vi "VisualizeNHRDC.vi"() -> ()   [LabVIEW 2018, in "Visualization.lvlib" / "VisualizeAcPwr.lvclass"]
doc: "This VI listens for any measurement data associated with the provided PluginName and displays it to the user for analysis. The display is only suitable for data coming from the NHR Battery Simulator Plugin."
uses:
  VisualizeAcPwr.lvclass
  VisualizeBase/VisualizeBase_class/Requests/VisUserEventType.ctl
  <vilib>/event_ctls.llb/usereventprio.ctl
  AcPwr/AcPwrShared/clMeasurmentData.ctl
  <vilib>/Analysis/baseanly.llb/Mean (DBL).vi
  <extravilib>/ChannelInstances/Tag-bool/Read With Abort.vi
  <extravilib>/ChannelInstances/Tag-bool/Write With Abort.vi
  <extravilib>/ChannelInstances/Tag-bool/Instantiate.vi
  <extravilib>/ChannelInstances/Tag-bool/EndpointRead.vi
  <vilib>/Utility/error.llb/Error Cluster From Error Code.vi
  <extravilib>/ChannelInstances/Tag-bool/Endpoint.vi
  <vilib>/ErrorRing/Error Ring.xnode
  VisualizeBase/VisualizeBase_class/VisualizeBase.lvclass
  <userlib>/NIST/NISTErrorLib/NISTErrorLib.lvlib
  <vilib>/Analysis/NI_AALBase.lvlib
  AcPwr/AcPwrShared/AcPwrShared.lvlib
  <extravilib>/ChannelInstances/Tag-bool.lvlib
panel:
  in  "Tab Control":enum32{"Chart", "XY Graph"}(tab)
  out "NHRDC":waveform(dbl)[](graph)=[{"t0"=timestamp(3657200531.6397257 s since 1904-01-01), "dt"=1.0, "Y"=[46.19]}, {"t0"=timestamp(3657200531.6397257 s since 1904-01-01), "dt"=1.0, "Y"=[2.0]}, {"t0"=timestamp(3657200531.6397257 s since 1904-01-01), "dt"=1.0, "Y"=[60.0]}]
  in  "PlotYAxis":u32[](array[numeric])=[0, 1, 0] max=1
  out "Incorrect DataType?":bool
  out "Current (A)":dbl(knob) scale=0.0..15.0
  out "Voltage (V)":dbl(knob) scale=0.0..100.0
  out "XY Graph":cluster{"Current":dbl[], "Voltage":dbl[]}[](graph)
  in  "Clear Graph":bool
  in  "PluginName":string="AcPwr.NHRDC0"
  out "ErrorArray":errorcluster[](array[cluster])
  in  "btnStop":bool
  in  "btnReset":bool
  in  "btnClear":bool
  # "0=Left Axis and 1=Right Axis"
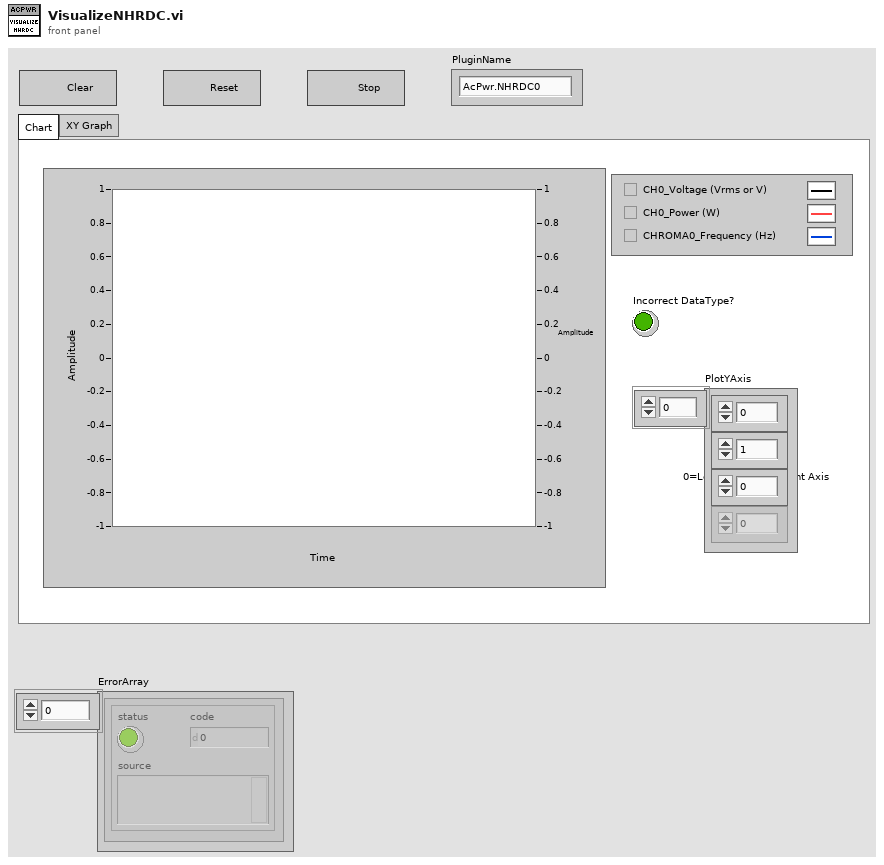
[diagram p1: front panel]
types:
  T1 = typedef "Visualization.lvlib/VisualizeBase.lvclass/VisRequestEvents.ctl" = cluster{"StopRequest":refnum<user-event>, "ResetRequest":refnum<user-event>, "FP Pop In or Out":refnum<user-event>}
  T2 = typedef "AcPwrShared.lvlib/AcPwrBroadcastEvents.ctl" = cluster{"DidInit":refnum<user-event>, "StatusUpdate":refnum<user-event>, "ErrorReport":refnum<user-event>, "DidStop":refnum<user-event>, "PathToINI":refnum<user-event>, "Measurements":refnum<user-event>, "LoadConfigFile":refnum<user-event>, "GetSettings":refnum<user-event>, "SetSettings":refnum<user-event>, "GetType&ID":refnum<user-event>, "GotSettings":refnum<user-event>}
  T3 = typedef "AcPwrShared.lvlib/clMeasurmentData.ctl" = cluster{"MeasName":string, "XML Data":string, "WaveformData":waveform(dbl)[]}
  T4 = typedef "Visualization.lvlib/VisualizeBase.lvclass/VisUserEventType.ctl" = cluster{"BusIndex":i8, "Data":variant}
  T5 = typedef "usereventprio.ctl" = enum32{"high priority", "normal priority"}
  T6 = typedef "Tag-bool.lvlib/))Channel.ctl" = refnum<queue>
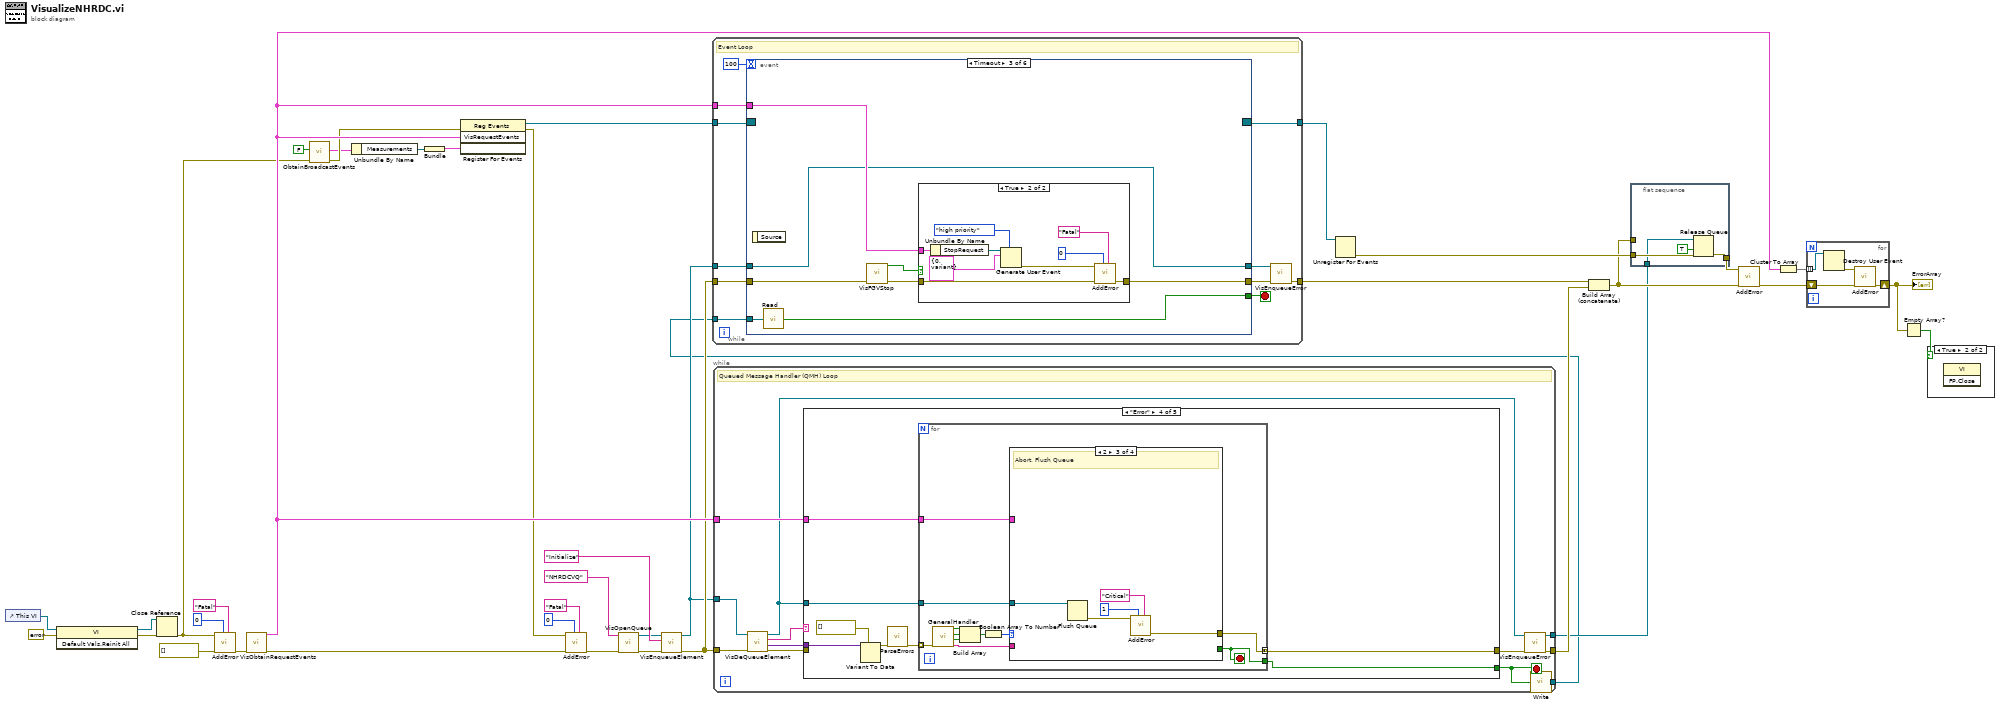
[diagram p0: block diagram]
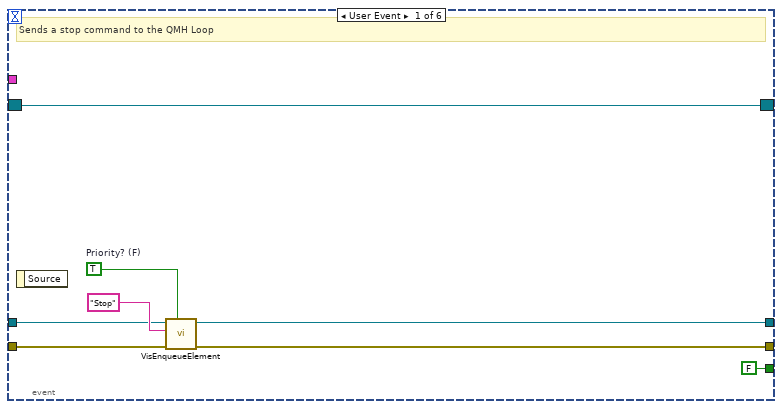
[diagram p2: hidden frame]
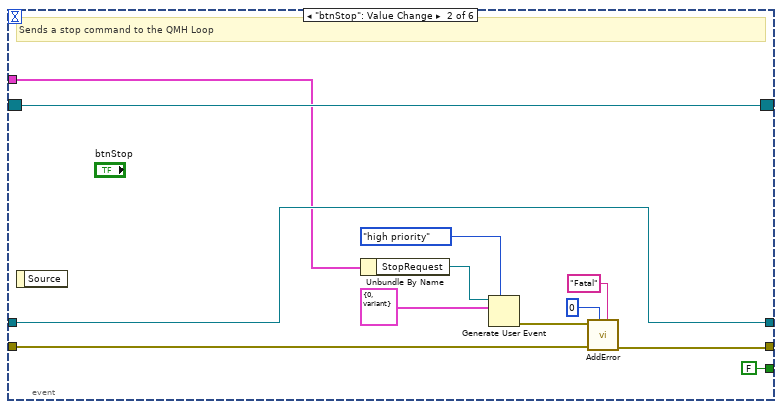
[diagram p3: hidden frame]
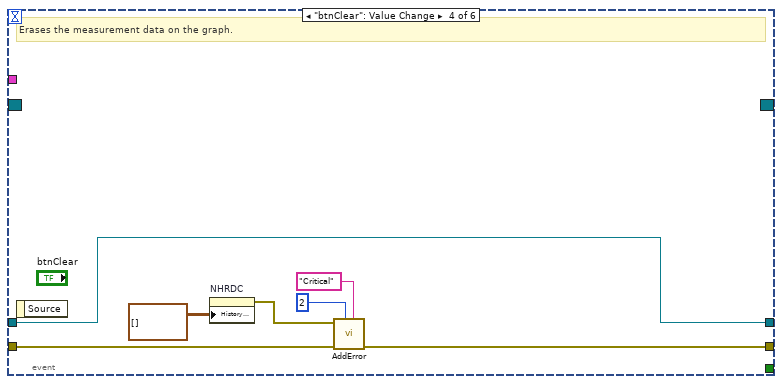
[diagram p5: hidden frame]
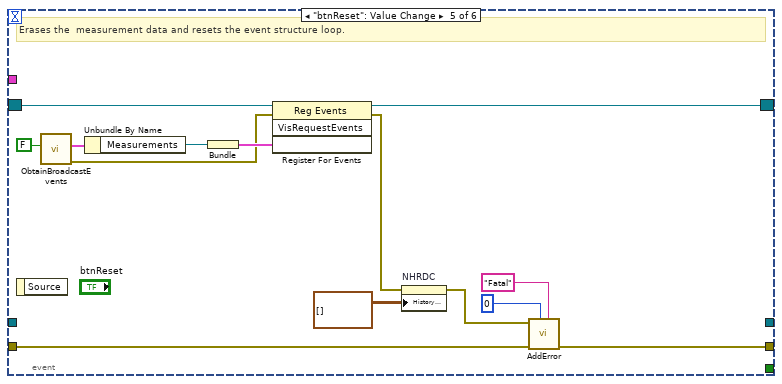
[diagram p6: hidden frame]
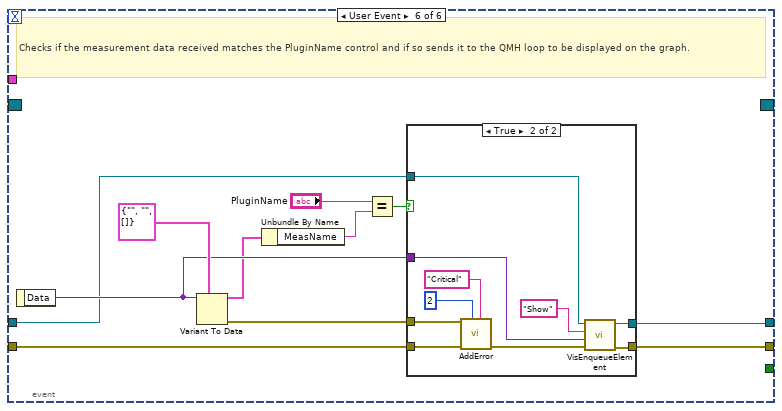
[diagram p7: hidden frame]
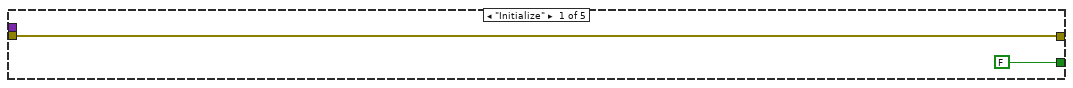
[diagram p9: hidden frame]
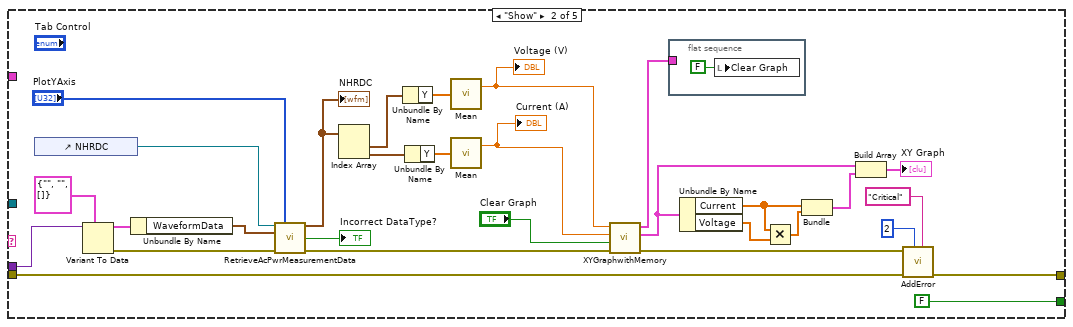
[diagram p10: hidden frame]
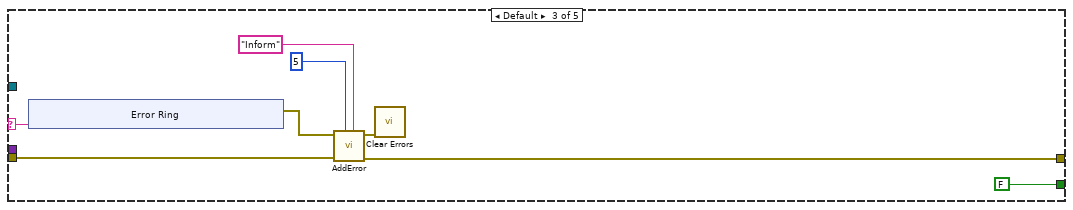
[diagram p11: hidden frame]
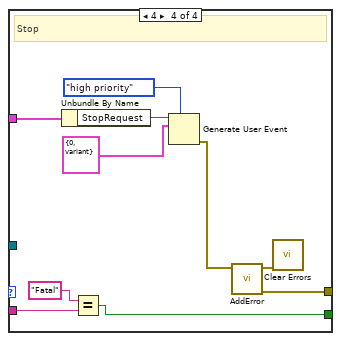
[diagram p14: hidden frame]
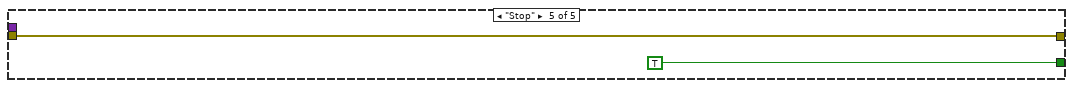
[diagram p15: hidden frame]
diagram:
  n1 = control-ref of="This VI"() -> (w26:refnum<vi>)
  n2 = invoke class="VI" method="Default Vals.Reinit All"(reference=w26, error in=errorcluster {"status"=FALSE, "code"=0, "source"=""} ("error in (no error)")) -> (reference out=w23:refnum<vi>, error out=w24:errorcluster)  [unwired: 1 in, 1 out]
  n3 = Close Reference(reference=w23, error in (no error)=w24) -> (error out=w21:errorcluster)
  n4 = call <userlib>:"AddError.vi"("Severity"="Fatal" ("String"), "Priority"=u8 0, "ErrorArray In"=errorcluster[] [] ("ErrorArray"), "error in (no error)"=w21) -> ("ErrorArray Out"=w38:errorcluster[])  [unwired: 6 in, 1 out]
  n5 = call "VisObtainRequestEvents.vi"("Error"=w38) -> ("Error"=w13:errorcluster[], "VisRequestEvents"=w30:T1)  [unwired: 9 in]
  n6 = call "ObtainBroadcastEvents.vi"("error in (no error)"=w21, "CreateNew? (F)"=FALSE) -> ("error out"=w20:errorcluster, "clAcPwrEvents"=w19:T2)  [unwired: 8 in]
  n7 = Unbundle By Name(w19) -> ("Measurements"=w28:refnum<user-event>)
  n8 = Bundle("Measurements"=w28) -> (w27:cluster{"Measurements":refnum<user-event>})  [unwired: 1 in]
  n9 = register-events(error in=w20, w30, w27) -> (reference out=w39:refnum<event-registration>, error out=w3:errorcluster)  [unwired: 1 in]
  n10 = call <userlib>:"AddError.vi"("Severity"="Fatal" ("String"), "Priority"=u8 0, "ErrorArray In"=w13, "error in (no error)"=w3) -> ("ErrorArray Out"=w10:errorcluster[])  [unwired: 6 in, 1 out]
  n11 = call "VisOpenQueue.vi"("Error Array In"=w10, "QueueName"="NHRDCVQ" ("QueuName")) -> ("Error Array Out"=w8:errorcluster[], "queue out"=w5:refnum<queue>)  [unwired: 8 in]
  n12 = call "VisEnqueueElement.vi"("Error Array In"=w8, "Message"="Initialize", "queue in"=w5) -> ("Error Array Out"=w7:errorcluster[], "queue out"=w4:refnum<queue>)  [unwired: 7 in]
  n13 = while {
    tunnel: w7 -> [w47]
    tunnel: [w49] -> w34
    tunnel: w30 -> [w48]
    tunnel: w4 -> [w46]
    tunnel: [w41] -> w2
    tunnel: [w40] -> w1
    stop <- w50 stop-if-true
    # "Queued Message Handler (QMH) Loop"
    n14 = call "VisDeQueueElement.vi"("Error Array In"=w47, "Queue In"=w46) -> ("Error Array Out"=w45:errorcluster[], "Data"=w44:variant, "Message"=w43:string, "Queue Out"=w42:refnum<queue>)  [unwired: 6 in]
    n15 = case shown="\"Error\"" w43 {
      selector: w43 -> [_ _ w92 _ _]
      tunnel: w44 -> [_ w79 _ w107 _]
      tunnel: w45 -> [w53 w80 w90 _ w134]
      tunnel: [w53 w83 w89 w103 w134] -> w51
      tunnel: [FALSE FALSE FALSE w102 TRUE] -> w50
      tunnel: w48 -> [_ _ _ w101 _]
      tunnel: w42 -> [_ _ _ w100 _]
      frame "Initialize" {
      }
      frame "Show" {
        n16 = control-ref of="NHRDC"() -> (w54:refnum<vi>)
        n17 = Variant To Data(type=T3 {"MeasName"="", "XML Data"="", "WaveformData"=[]} ("MeasurmentDataCluster"), Variant=w79) -> (data=w58:T3, error out=w61:errorcluster)  [unwired: 1 in]
        n18 = Unbundle By Name(w58) -> ("WaveformData"=w57:waveform(dbl)[])
        n19 = call "RetrieveAcPwrMeasurementData.vi"("WaveformChartReference"=w54, "PlotYScale"="PlotYAxis", "WaveformArrayIn"=w57, "error in (no error)"=w61) -> ("WaveformArrayOut"=w55:waveform(dbl)[], "Incorrect DataType?"=→"Incorrect DataType?":bool, "error out"=w60:errorcluster)  [unwired: 7 in, 2 out]
        "NHRDC" <- w55
        n20 = Index Array(array=w55) -> (element #1=w78:waveform(dbl), element #2=w77:waveform(dbl))  [unwired: 2 in]
        n21 = Unbundle By Name(w78) -> ("Y"=w75:dbl[])
        n22 = Unbundle By Name(w77) -> ("Y"=w74:dbl[])
        n23 = call-poly <vilib>:"Mean.vi"("X"=w75) -> ("mean"=w72:dbl)  [unwired: 1 out]
        "Voltage (V)" <- w72
        n24 = call-poly <vilib>:"Mean.vi"("X"=w74) -> ("mean"=w70:dbl)  [unwired: 1 out]
        "Current (A)" <- w70
        n25 = call "XYGraphwithMemory.vi"("Error In"=w60, "Clear Graph"="Clear Graph", "Current"=w70, "Voltage"=w72) -> ("Error Out"=w71:errorcluster, "output cluster"=w68:cluster{"Current":dbl[], "Voltage":dbl[]}, "Cluster"=w69:cluster{"Array":dbl[], "Array":dbl[]})  [unwired: 5 in]
        n26 = flat-sequence {
          tunnel: w69 -> [_]
          frame #0 {
            n27 = local write "Clear Graph"(FALSE ("Clear Graph")) -> ()
          }
        }
        n28 = Unbundle By Name(w68) -> ("Current"=w64:dbl[], "Voltage"=w65:dbl[])
        n29 = Multiply(x=w64, y=w65) -> (x*y=w63:dbl[])
        n30 = Bundle("Current"=w64, w63) -> (w66:cluster{"Current":dbl[], dbl[]})  [unwired: 1 in]
        n31 = Build Array(w68, w66) -> (→"XY Graph":cluster{"Current":dbl[], "Voltage":dbl[]}[])
        n32 = call <userlib>:"AddError.vi"("Severity"="Critical" ("String"), "Priority"=u8 2, "ErrorArray In"=w80, "error in (no error)"=w71) -> ("ErrorArray Out"=w83:errorcluster[])  [unwired: 6 in, 1 out]
      }
      frame Default {
        n33 = xnode "Error Ring"("parameter 0"=w92) -> ("error out"=w91:errorcluster)
        n34 = call <userlib>:"AddError.vi"("Severity"="Inform" ("String"), "Priority"=u8 5, "ErrorArray In"=w90, "error in (no error)"=w91) -> ("ErrorArray Out"=w89:errorcluster[], "error out"=w88:errorcluster)  [unwired: 6 in]
        n35 = call <vilib>:"Clear Errors.vi"("error in (no error)"=w88) -> ()  [unwired: 5 in, 2 out]
      }
      frame "Error" {
        n36 = Variant To Data(type=errorcluster[] [], Variant=w107) -> (data=w105:errorcluster[])  [unwired: 1 in, 1 out]
        n37 = call <userlib>:"ParseErrors.vi"("ErrorArray"=w105) -> ("ErrorArray"=w104:errorcluster[])  [unwired: 8 in, 2 out]
        n38 = for {
          tunnel: w104 -> [w118] mode=indexing
          tunnel: [w112] -> w103 mode=concatenating
          tunnel: [w110] -> w102
          tunnel: w101 -> [w109]
          tunnel: w100 -> [w108]
          stop <- w110 stop-if-true
          n39 = call <userlib>:"GeneralHandler.vi"("error in (no error)"=w118) -> ("Severity"=w111:string, "Stop"=w115:bool, "Abort"=w116:bool, "Continue"=w117:bool)  [unwired: 6 in, 1 out]
          n40 = Build Array(w117, w116, w115) -> (w114:bool[])
          n41 = Boolean Array To Number(Boolean array=w114) -> (number=w113:u32)
          n42 = case shown="2" w113 {
            tunnel: [_ _ w123 w132] -> w112
            tunnel: w111 -> [_ _ _ w127]
            tunnel: [_ _ _ w125] -> w110
            tunnel: w109 -> [_ _ _ w124]
            tunnel: w108 -> [_ _ w119 _]
            frame 0, Default {
              # "No Dialog"
            }
            frame 1 {
              # "Continue"
            }
            frame 2 {
              # "Abort, Flush Queue"
              n43 = Flush Queue(queue=w119) -> (error out=w122:errorcluster)  [unwired: 1 in, 2 out]
              n44 = call <userlib>:"AddError.vi"("Severity"="Critical" ("String"), "Priority"=u8 1, "error in (no error)"=w122) -> ("ErrorArray Out"=w123:errorcluster[])  [unwired: 7 in, 1 out]
            }
            frame 4 {
              # "Stop"
              n45 = Unbundle By Name(w124) -> ("StopRequest"=w133:refnum<user-event>)
              n46 = Equal?(x="Fatal", y=w127) -> (x = y?=w125:bool)
              n47 = Generate User Event(priority (normal)=usereventprio."high priority", user event=w133, event data cluster=T4 {"BusIndex"=0, "Data"=variant} ("event data")) -> (error out=w131:errorcluster)  [unwired: 1 in, 1 out]
              n48 = call <userlib>:"AddError.vi"("error in (no error)"=w131) -> ("ErrorArray Out"=w132:errorcluster[], "error out"=w128:errorcluster)  [unwired: 9 in]
              n49 = call <vilib>:"Clear Errors.vi"("error in (no error)"=w128) -> ()  [unwired: 5 in, 2 out]
            }
          }
        }
      }
      frame "Stop" {
      }
    }
    n50 = call "VisEnqueueError.vi"("Error Array In"=w51, "Queue in"=w42) -> ("Error Array Out"=w49:errorcluster[], "Queue out"=w41:refnum<queue>)  [unwired: 8 in]
    n51 = call <extravilib>:"Write.vi"("element"=w50) -> ("channel"=w40:T6)  [unwired: 1 out]
  }
  n52 = while {
    tunnel: w39 -> [w146]
    tunnel: [w143] -> w35
    tunnel: [w142] -> w37
    tunnel: w30 -> [w141]
    tunnel: w7 -> [w140]
    tunnel: w4 -> [w139]
    tunnel: w1 -> [w136]
    stop <- w145 stop-if-true
    # "Event Loop"
    n53 = event shown="[2] Timeout" {
      selector: w146 -> [w148 w156 _ _ w205 _]
      dyn-events: [w148 w156 _ _ w204 _] -> w142
      timeout: 100 -> [_ _ _ _ _ _]
      tunnel: [FALSE FALSE w167 _ _ _] -> w145
      tunnel: [w149 w157 w169 w189 w199 w216] -> w144
      tunnel: w141 -> [_ w155 w171 _ _ _]
      tunnel: w140 -> [w152 w166 w172 w188 w198 w214]
      tunnel: w139 -> [w151 w165 w170 w185 _ w207]
      tunnel: [w147 w165 w170 w185 _ w206] -> w138
      tunnel: w136 -> [_ _ w168 _ _ _]
      event User Event {
        w153 = TRUE  # Priority? (F)
        # "Sends a stop command to the QMH Loop"
        n54 = event-data() -> ()  [unwired: 1 in, 1 out]
        n55 = call "VisEnqueueElement.vi"("Priority? (F)"=w153, "Error Array In"=w152, "Message"="Stop", "queue in"=w151) -> ("Error Array Out"=w149:errorcluster[], "queue out"=w147:refnum<queue>)  [unwired: 6 in]
      }
      event "btnStop": Value Change {
        # "Sends a stop command to the QMH Loop"
        n56 = event-data() -> ()  [unwired: 1 in, 1 out]
        n57 = Unbundle By Name(w155) -> ("StopRequest"=w162:refnum<user-event>)
        n58 = Generate User Event(priority (normal)=usereventprio."high priority", user event=w162, event data cluster=T4 {"BusIndex"=0, "Data"=variant} ("event data")) -> (error out=w163:errorcluster)  [unwired: 1 in, 1 out]
        n59 = call <userlib>:"AddError.vi"("Severity"="Fatal" ("String"), "Priority"=u8 0, "ErrorArray In"=w166, "error in (no error)"=w163) -> ("ErrorArray Out"=w157:errorcluster[])  [unwired: 6 in, 1 out]
      }
      event Timeout {
        n60 = event-data() -> ()  [unwired: 1 in, 1 out]
        n61 = call <extravilib>:"Read.vi"("channel"=w168) -> ("element"=w167:bool)  [unwired: 1 in, 1 out]
        n62 = call "VisFGVStop.vi"("Error In"=w172) -> ("Error Out"=w173:errorcluster[], "Value"=w174:bool)  [unwired: 9 in]
        n63 = case shown="True" w174 {
          tunnel: w173 -> [w175 w184]
          tunnel: [w175 w177] -> w169
          tunnel: w171 -> [_ w176]
          frame False {
          }
          frame True {
            n64 = Unbundle By Name(w176) -> ("StopRequest"=w182:refnum<user-event>)
            n65 = Generate User Event(priority (normal)=usereventprio."high priority", user event=w182, event data cluster=T4 {"BusIndex"=0, "Data"=variant} ("event data")) -> (error out=w183:errorcluster)  [unwired: 1 in, 1 out]
            n66 = call <userlib>:"AddError.vi"("Severity"="Fatal" ("String"), "Priority"=u8 0, "ErrorArray In"=w184, "error in (no error)"=w183) -> ("ErrorArray Out"=w177:errorcluster[])  [unwired: 6 in, 1 out]
          }
        }
      }
      event "btnClear": Value Change {
        # "Erases the measurement data on the graph."
        n67 = event-data() -> ()  [unwired: 1 in, 1 out]
        n68 = property on="NHRDC" class="WFChart (strict)"("History Data"=waveform(dbl)[][] []) -> (error out=w186:errorcluster)  [unwired: 2 in, 1 out]
        n69 = call <userlib>:"AddError.vi"("Severity"="Critical" ("String"), "Priority"=u8 2, "ErrorArray In"=w188, "error in (no error)"=w186) -> ("ErrorArray Out"=w189:errorcluster[])  [unwired: 6 in, 1 out]
      }
      event "btnReset": Value Change {
        # "Erases the  measurement data and resets the event structure loop."
        n70 = event-data() -> ()  [unwired: 1 in, 1 out]
        n71 = call "ObtainBroadcastEvents.vi"("CreateNew? (F)"=FALSE) -> ("error out"=w200:errorcluster, "clAcPwrEvents"=w201:T2)  [unwired: 9 in]
        n72 = Unbundle By Name(w201) -> ("Measurements"=w203:refnum<user-event>)
        n73 = Bundle("Measurements"=w203) -> (w202:cluster{"Measurements":refnum<user-event>})  [unwired: 1 in]
        n74 = register-events(reference=w205, error in=w200, w202) -> (reference out=w204:refnum<event-registration>, error out=w194:errorcluster)  [unwired: 1 in]
        n75 = property on="NHRDC" class="WFChart (strict)"(error in=w194, "History Data"=waveform(dbl)[][] []) -> (error out=w195:errorcluster)  [unwired: 1 in, 1 out]
        n76 = call <userlib>:"AddError.vi"("Severity"="Fatal" ("String"), "Priority"=u8 0, "ErrorArray In"=w198, "error in (no error)"=w195) -> ("ErrorArray Out"=w199:errorcluster[])  [unwired: 6 in, 1 out]
      }
      event User Event {
        # "Checks if the measurement data received matches the PluginName control and if so sends it to the QMH loop to be displayed on the graph."
        n77 = event-data() -> ("Data"=w210:variant)  [unwired: 1 in]
        n78 = Variant To Data(type=T3 {"MeasName"="", "XML Data"="", "WaveformData"=[]} ("MeasurmentDataCluster"), Variant=w210) -> (data=w209:T3, error out=w213:errorcluster)  [unwired: 1 in]
        n79 = Unbundle By Name(w209) -> ("MeasName"=w208:string)
        n80 = Equal?(x="PluginName", y=w208) -> (x = y?=w215:bool)
        n81 = case shown="True" w215 {
          tunnel: [w218 w227] -> w216
          tunnel: w214 -> [w218 w223]
          tunnel: w210 -> [_ w226]
          tunnel: w213 -> [_ w221]
          tunnel: w207 -> [w217 w220]
          tunnel: [w217 w219] -> w206
          frame False {
          }
          frame True {
            n82 = call <userlib>:"AddError.vi"("Severity"="Critical" ("String"), "Priority"=u8 2, "ErrorArray In"=w223, "error in (no error)"=w221) -> ("ErrorArray Out"=w222:errorcluster[])  [unwired: 6 in, 1 out]
            n83 = call "VisEnqueueElement.vi"("Error Array In"=w222, "Data"=w226, "Message"="Show", "queue in"=w220) -> ("Error Array Out"=w227:errorcluster[], "queue out"=w219:refnum<queue>)  [unwired: 6 in]
          }
        }
      }
    }
    n84 = call "VisEnqueueError.vi"("Error Array In"=w144, "Queue in"=w138) -> ("Error Array Out"=w143:errorcluster[])  [unwired: 8 in, 1 out]
  }
  n85 = Unregister For Events(event registration refnum=w37) -> (error out=w33:errorcluster)  [unwired: 1 in]
  n86 = Build Array (concatenate)(w35, w34) -> (w12:errorcluster[])
  n87 = flat-sequence {
    tunnel: w33 -> [w232]
    tunnel: [w231] -> w32
    tunnel: w12 -> [_]
    tunnel: w2 -> [w230]
    frame #0 {
      n88 = Release Queue(queue=w230, force destroy? (F)=TRUE, error in (no error)=w232) -> (error out=w231:errorcluster)  [unwired: 2 out]
    }
  }
  n89 = call <userlib>:"AddError.vi"("ErrorArray In"=w12, "error in (no error)"=w32) -> ("ErrorArray Out"=w31:errorcluster[])  [unwired: 8 in, 1 out]
  n90 = Cluster To Array(cluster=w30) -> (array=w36:refnum<user-event>[])
  n91 = for {
    tunnel: w36 -> [w236] mode=indexing
    shift-right: [w235] -> w22
    shift-left: w31 -> [w234]
    n92 = Destroy User Event(user event=w236) -> (error out=w233:errorcluster)  [unwired: 1 in]
    n93 = call <userlib>:"AddError.vi"("ErrorArray In"=w234, "error in (no error)"=w233) -> ("ErrorArray Out"=w235:errorcluster[])  [unwired: 8 in, 1 out]
  }
  "ErrorArray" <- w22
  n94 = Empty Array?(array=w22) -> (empty?=w29:bool)
  n95 = case shown="True" w29 {
    frame False {
    }
    frame True {
      n96 = invoke class="VI" method="FP.Close"() -> ()  [unwired: 3 in, 3 out]
    }
  }
